vi "test_Write I64 Register Value.vi"(8 "error in (no error)":errorcluster, 11 "TestCase in":refnum<class "FPGA Register IO Tests.lvclass">) -> (0 "error out":errorcluster, 3 "TestCase out":refnum<class "FPGA Register IO Tests.lvclass">)   [LabVIEW 2020, in "FPGA Register IO Tests.lvclass"]
uses:
  FPGA Register IO Tests.lvclass
  FPGA Register IO Tests.lvclass/FPGA Register IO Tests.ctl
  APIs/FPGA Register IO/Write Methods/Write Data Register/Instances/Write I64.vi
  APIs/FPGA Register IO/Read Methods/Read Data Register/Instances/Read I64.vi
  APIs/FPGA Register IO/Utilities/Find Register Offset.vi
  APIs/FPGA Register IO/SubVIs/Check Register Data Store.vi
  APIs/FPGA Register IO/Error Handling/Error 6001.vi
  APIs/FPGA Register IO/Error Handling/Error 6000.vi
  APIs/FPGA Register IO/Error Handling/Error 6002.vi
  APIs/FPGA Register IO/Error Handling/Error 6006.vi
  APIs/FPGA Register IO/Error Handling/Error 6003.vi
  <vilib>/FPGAPlugInAG/Dynamic/niLvFpga_Close_Dynamic.vi
  <vilib>/rvi/interface/nirviCloseFPGA/nirviCloseFPGA.xnode
  <vilib>/addons/_JKI Toolkits/VI Tester/TestCase.llb/TestCase.lvclass
  APIs/FPGA Register IO/FPGA Register IO.lvlib
  C:/Program Files (x86)/National Instruments/LabVIEW 2020/vi.lib/addons/_JKI Toolkits/VI Tester/TestCase.llb/TestCase.lvclass
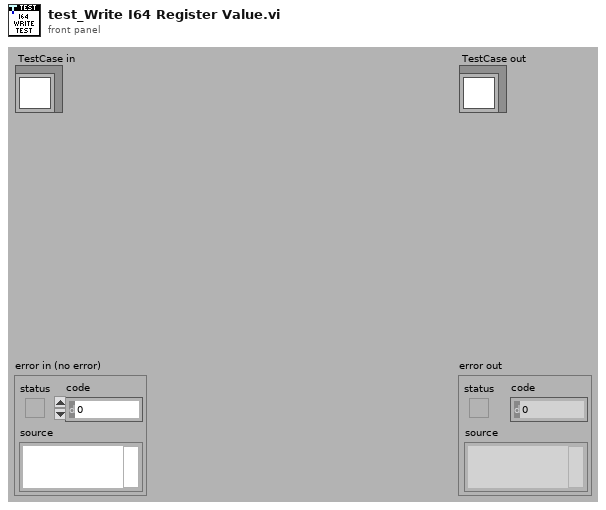
[diagram p1: front panel]
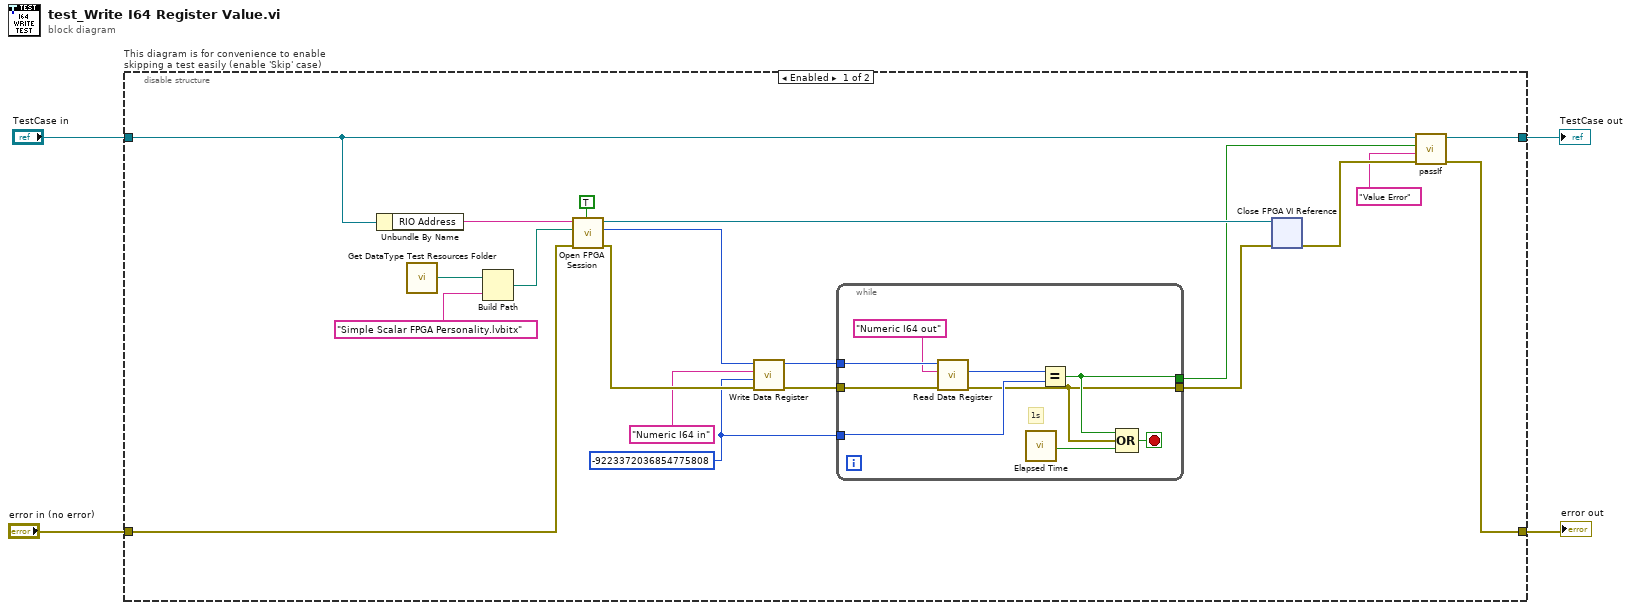
[diagram p0: block diagram]
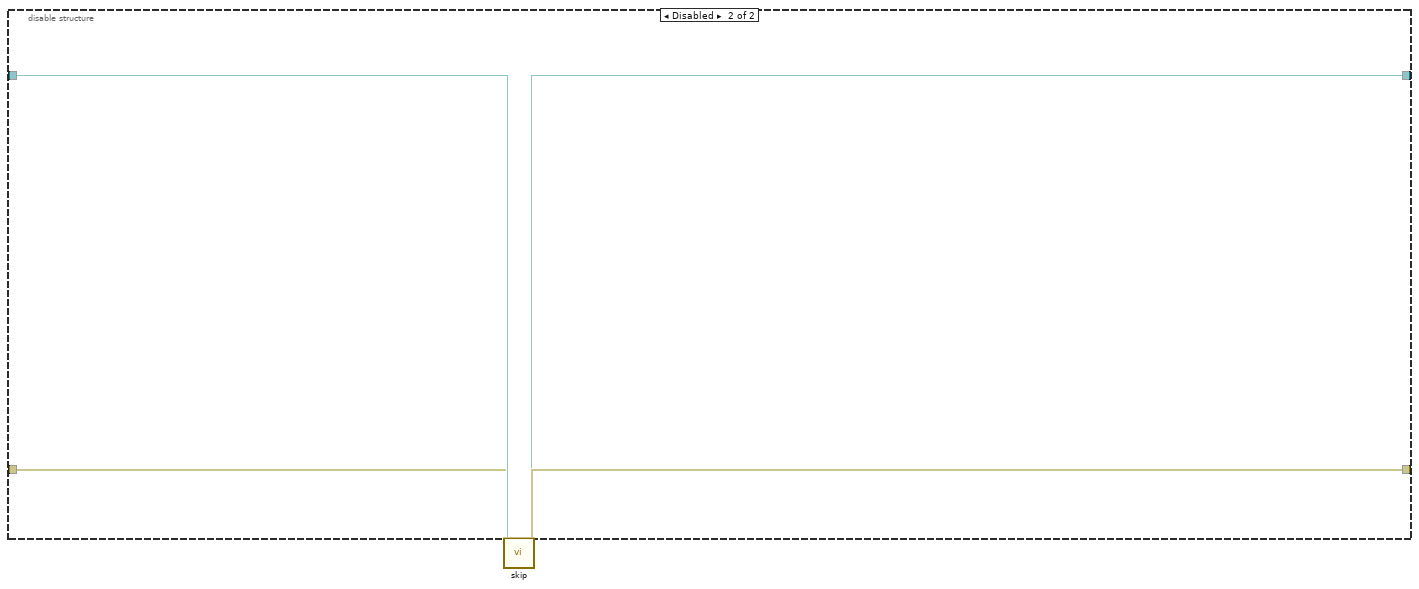
[diagram p2: hidden frame]
diagram:
  n1 = disable-structure "This diagram is for convenience to enable skipping a test easily (enable 'Skip' case)" shown="Enabled" {
    disable-tunnel: "TestCase in" -> [w19 w37]
    disable-tunnel: [w15 w35] -> w1
    disable-tunnel: [w14 w36] -> w3
    disable-tunnel: "error in (no error)" -> [w20 w34]
    frame Enabled {
      w7 = i64 -9223372036854775808 ("value in")
      n2 = Unbundle By Name(w19) -> ("RIO Address"=w13:string)
      n3 = call "Get DataType Test Resources Folder.vi"() -> ("path"=w17:path)
      n4 = Build Path(base path=w17, name or relative path="Simple Scalar FPGA Personality.lvbitx") -> (appended path=w21:path)
      n5 = call "Open FPGA Session.vi"("run when loaded (T)"=TRUE ("Run When Loaded (T)"), "error in"=w20, "bitfile path"=w21, "device address"=w13) -> ("error out"=w12:errorcluster, "session out"=w10:u32, "bitfile reference out"=w23:refnum<k20>)  [unwired: 5 in]
      n6 = call-poly "Write Data Register.vi"("error in"=w12, "value in"=w7, "register name"="Numeric I64 in", "session in"=w10) -> ("error out"=w8:errorcluster, "session out"=w9:u32)  [unwired: 6 in]
      n7 = while {
        tunnel: [w27] -> w6
        tunnel: w8 -> [w33]
        tunnel: w9 -> [w32]
        tunnel: w7 -> [w31]
        tunnel: [w28] -> w5
        stop <- w29 stop-if-true
        # "1s"
        n8 = call-poly "Read Data Register.vi"("error in"=w33, "register name"="Numeric I64 out", "session in"=w32) -> ("error out"=w27:errorcluster, "value out"=w30:i64)  [unwired: 6 in, 1 out]
        n9 = call "Elapsed Time"() -> ("Time has Elapsed"=w26:bool)  [unwired: 12 in, 7 out]
        n10 = Equal?(x=w30, y=w31) -> (x = y?=w28:bool)
        n11 = Compound Arithmetic op=OR(w28, w27, w26) -> (w29:bool)
      }
      n12 = xnode "Close FPGA VI Reference"("FPGA VI Reference In"=w23, "error in"=w6) -> ("error out"=w18:errorcluster)
      n13 = call-dynamic "passIf.vi"("error in (no error)"=w18, "message (\"\")"="Value Error" ("message (\"\")"), "pass"=w5, "TestCase in"=w19) -> ("error out"=w14:errorcluster, "TestCase out"=w15:refnum<class "FPGA Register IO Tests.lvclass">)  [unwired: 6 in]
    }
    frame Disabled {
      # "skip test result while test is under development"
      n14 = call <vilib>:"skip.vi"("error in (no error)"=w34, "TestCase in"=w37) -> ("error out"=w36:errorcluster, "TestCase out"=w35:refnum<class "FPGA Register IO Tests.lvclass">)  [unwired: 8 in]
    }
  }
  "error out" <- w3
  "TestCase out" <- w1
